vi "Insert Error.Record.vi"(8 "error in (no error)":errorcluster, 11 "Error":T1) -> (0 "error out":errorcluster)   [LabVIEW 2017, in "SQLite.lvclass"]
doc: "更新Limitation表格里面的Min和Max，根据输入的不同而更新不同的内容。\nValue 的输入必须最少包含Min和Max的值。\n\n2015-11-03 10:20:20\n蒋松\njiangsong@outlook.com"
uses:
  SQLite.lvclass
  Error Details.ctl
  SQLiteFileName.ctl
  TabelFullName.ctl
  <vilib>/Utility/error.llb/Trim Whitespace.vi
  <userlib>/sushu/sushu.lvlib
  <userlib>/LabSQL/LabSQL.lvlib
panel:
  in  "VI Ref":refnum<vi>
  in  "Alarm?":bool=TRUE
  in  "CMD":T2(ring)=enum."Read"
  out "array":string[](array[string])
  out "concatenated string":string
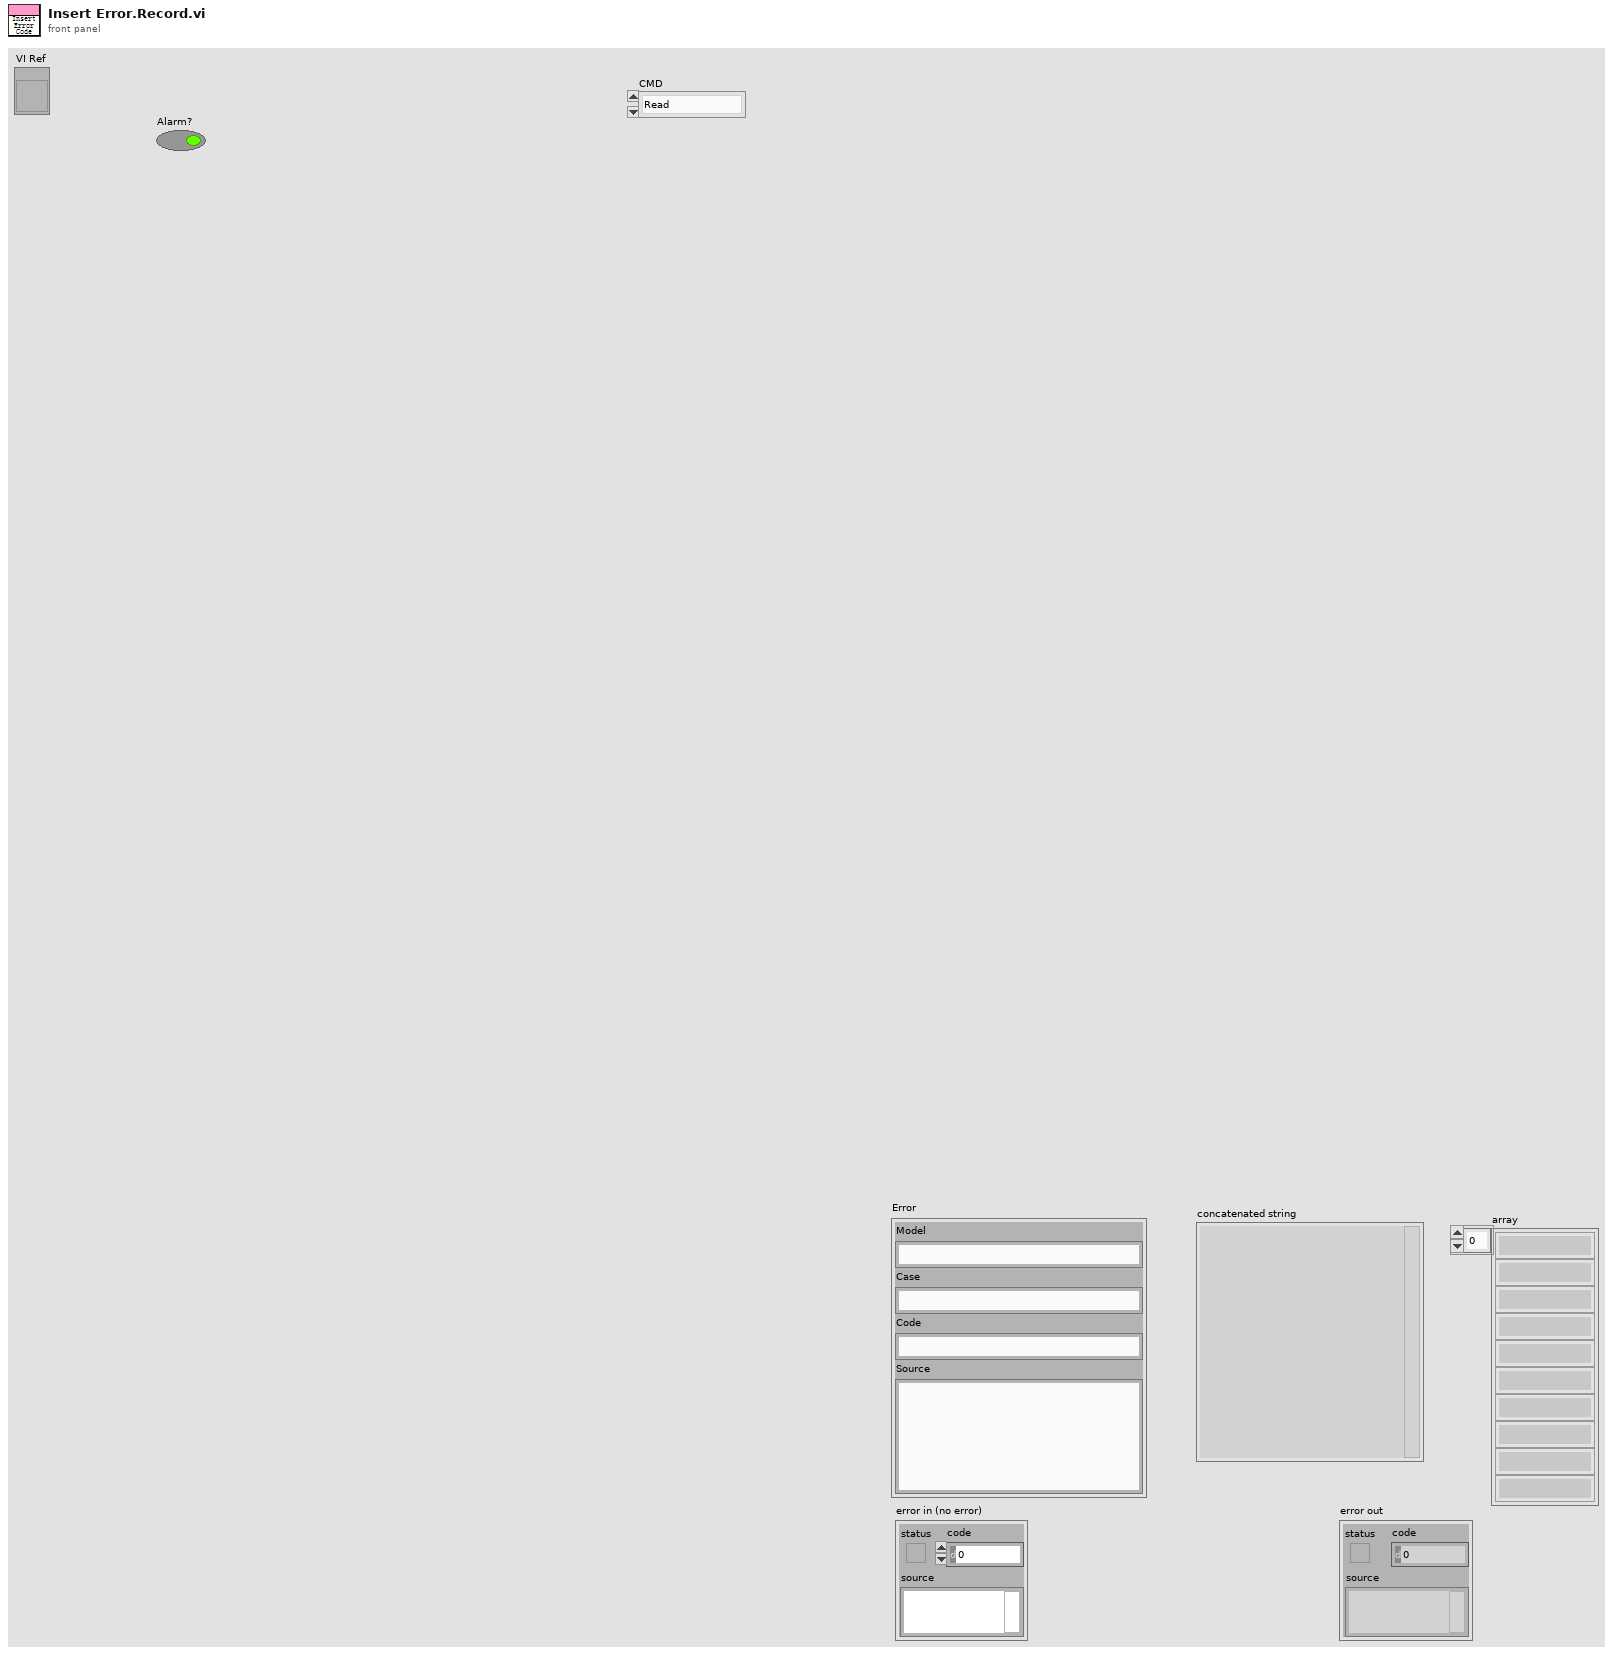
[diagram p1: front panel]
types:
  T1 = typedef "SQLite.lvclass/Error Details.ctl" = cluster{"Model":string, "Case":string, "Code":string, "Source":string}
  T2 = enum16{"Initialize", "Read", "Write", "UnInitialize"}
  T3 = typedef "SQLite.lvclass/TabelFullName.ctl" = string
  T4 = typedef "SQLite.lvclass/SQLiteFileName.ctl" = string
  T5 = cluster{"Current VI Reference":refnum<vi>, "Close Panel on Exit?":bool}
  T6 = cluster{"Core":cluster{"Current VI Reference":refnum<vi>, "Close Panel on Exit?":bool}, "VI Name":string}
  T7 = enum32{"invalid app kind", "Development System", "Run Time System", "Student Edition", "Embedded LabVIEW", "Evaluation", "Custom"}
  T8 = enum32{"Invalid", "Standard", "Closed", "Hidden", "Minimized", "Maximized"}
  T9 = enum16{"Other", "SQL2008", "SQLite", "Access", "MySQL"}
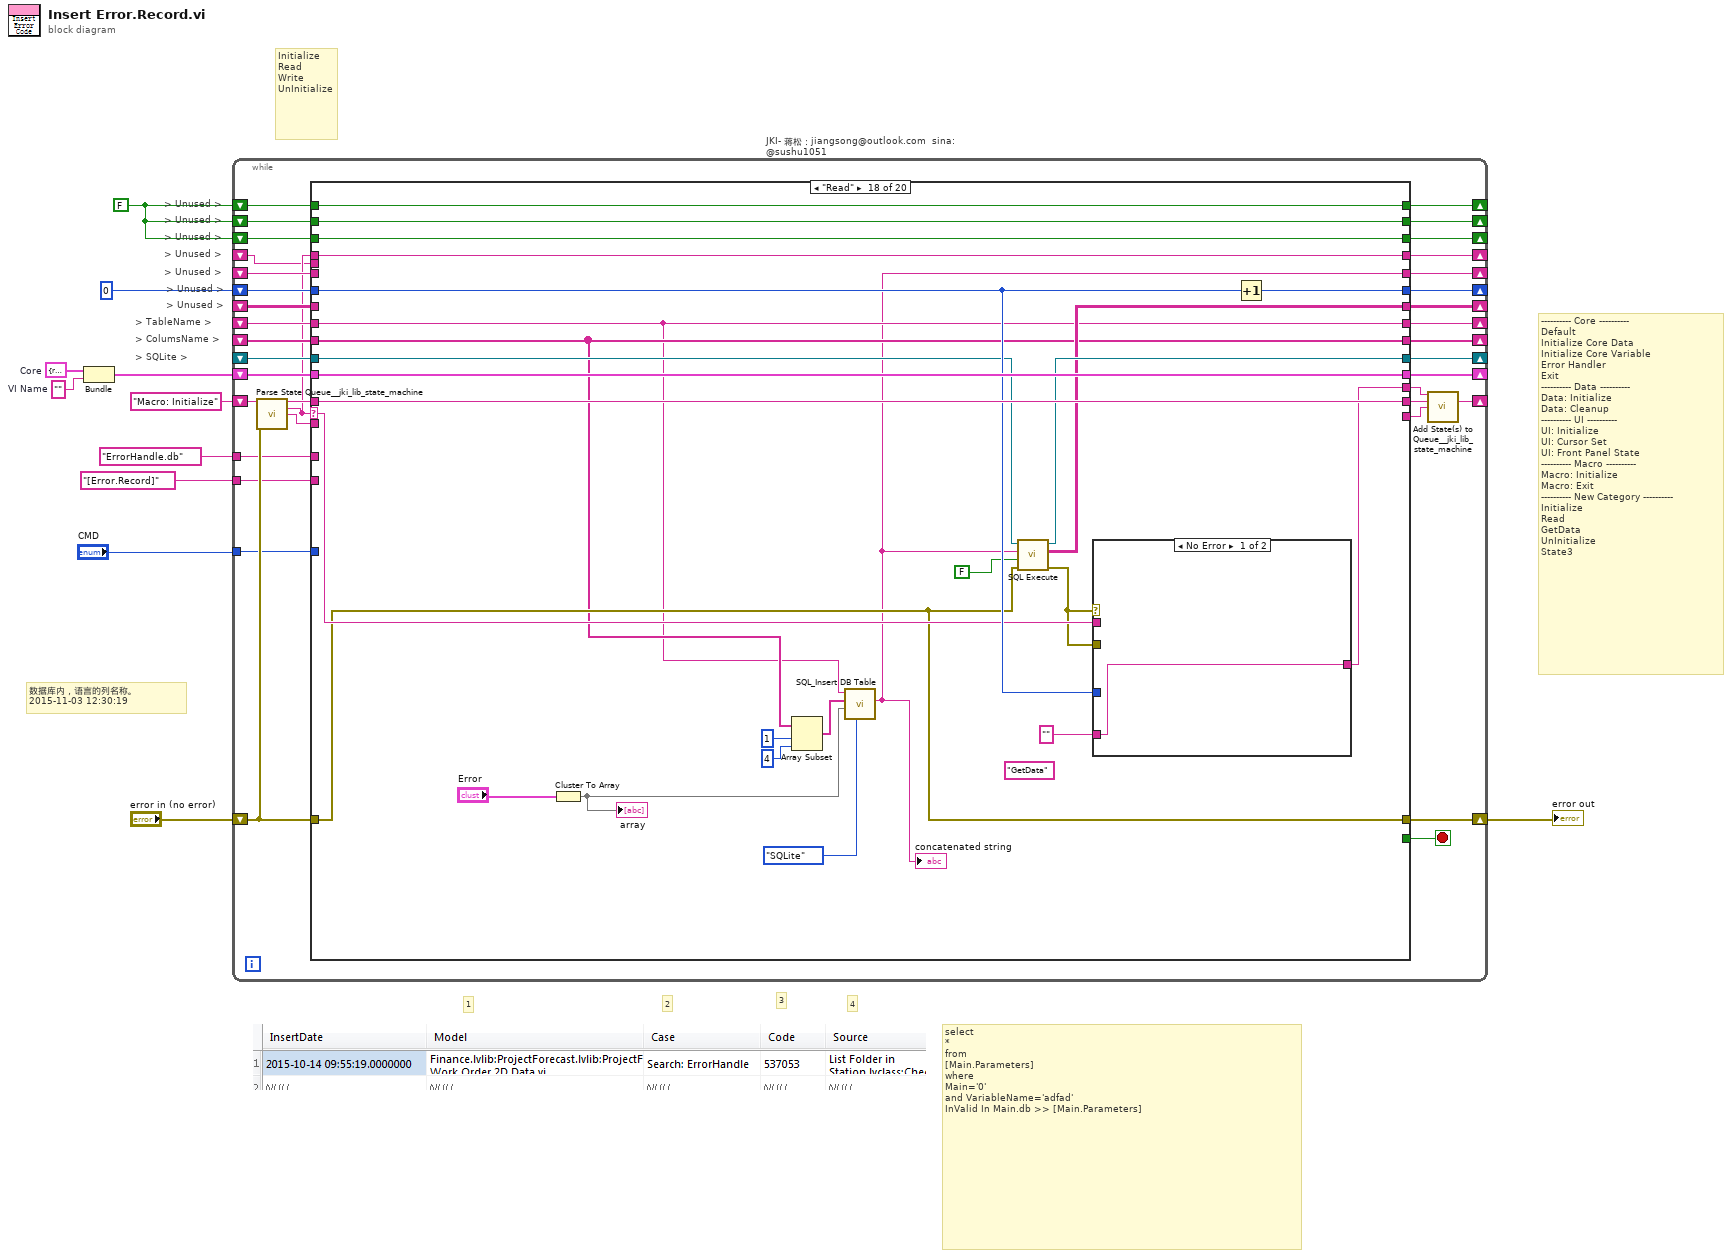
[diagram p0: block diagram]
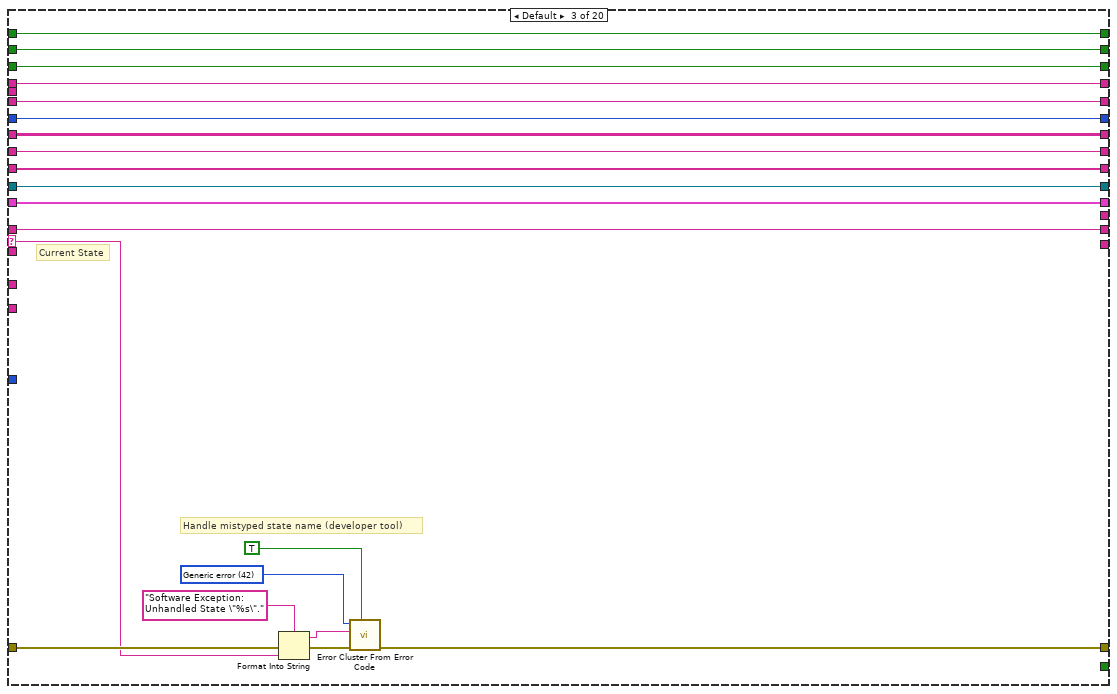
[diagram p4: hidden frame]
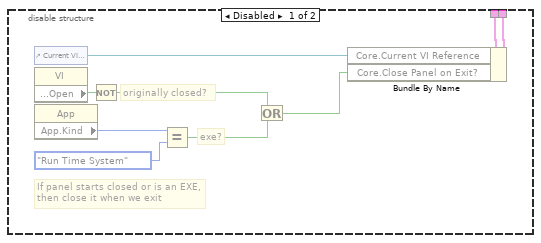
[diagram p6: hidden frame]
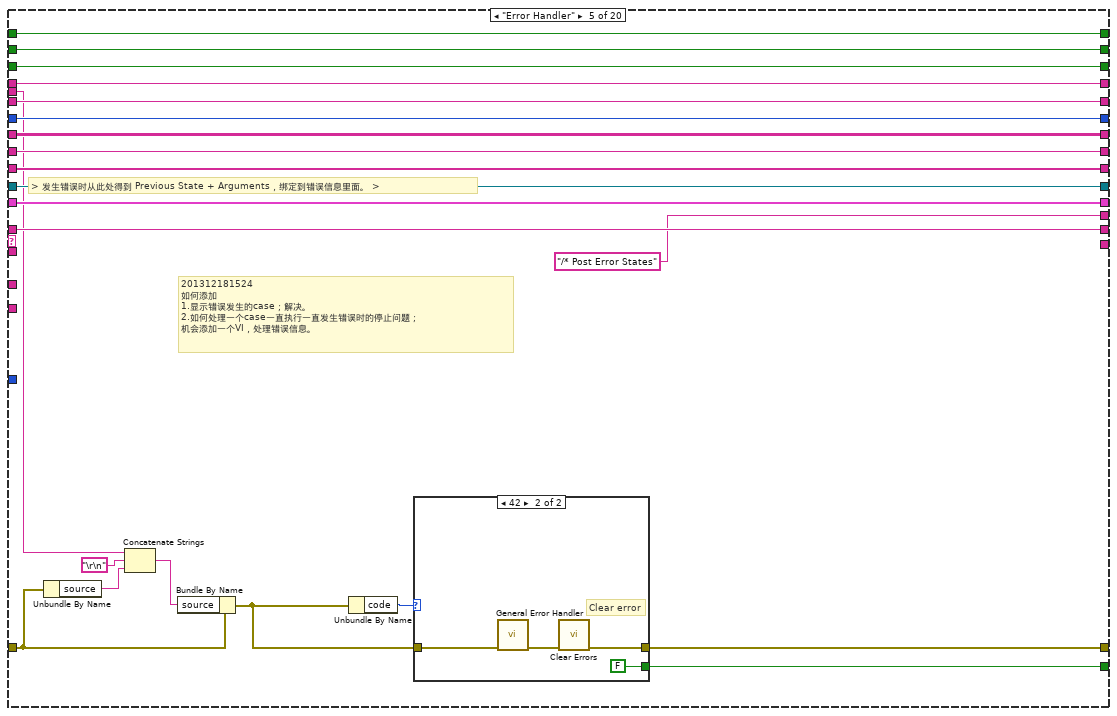
[diagram p7: hidden frame]
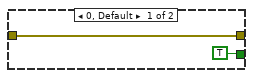
[diagram p8: hidden frame]
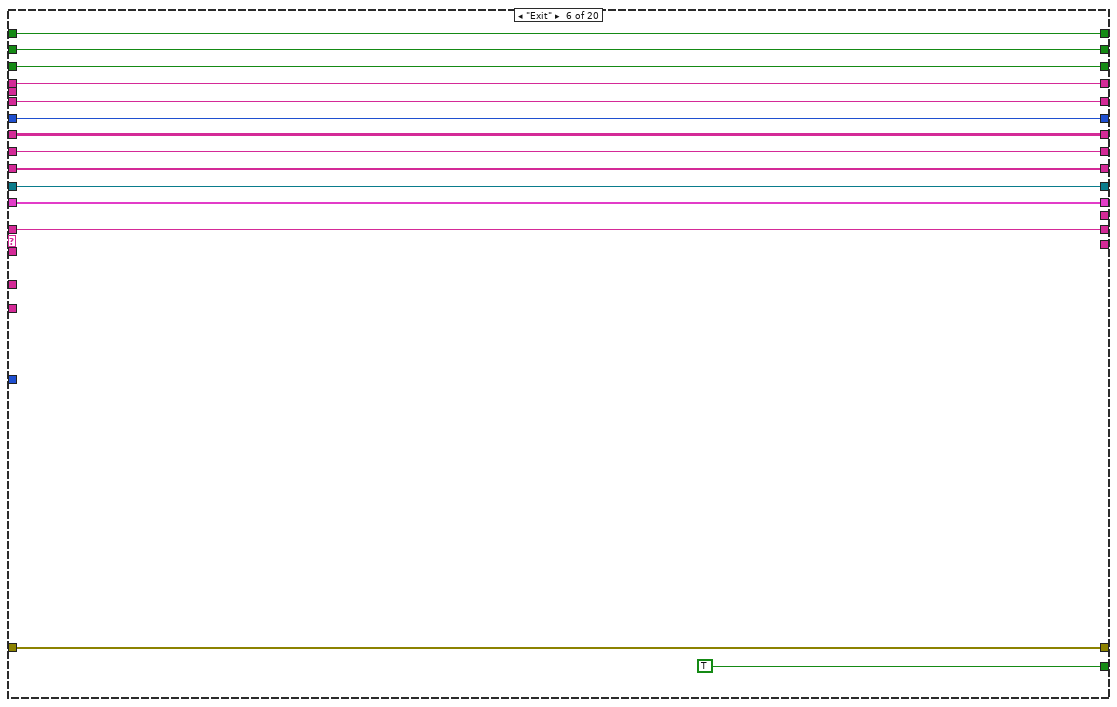
[diagram p9: hidden frame]
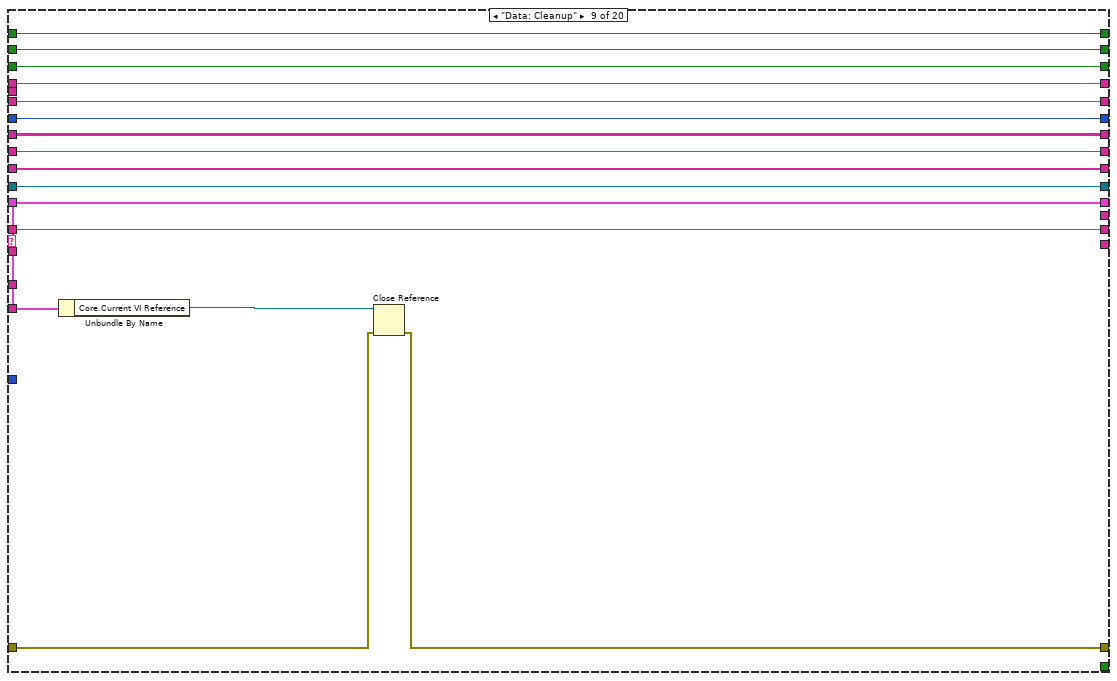
[diagram p12: hidden frame]
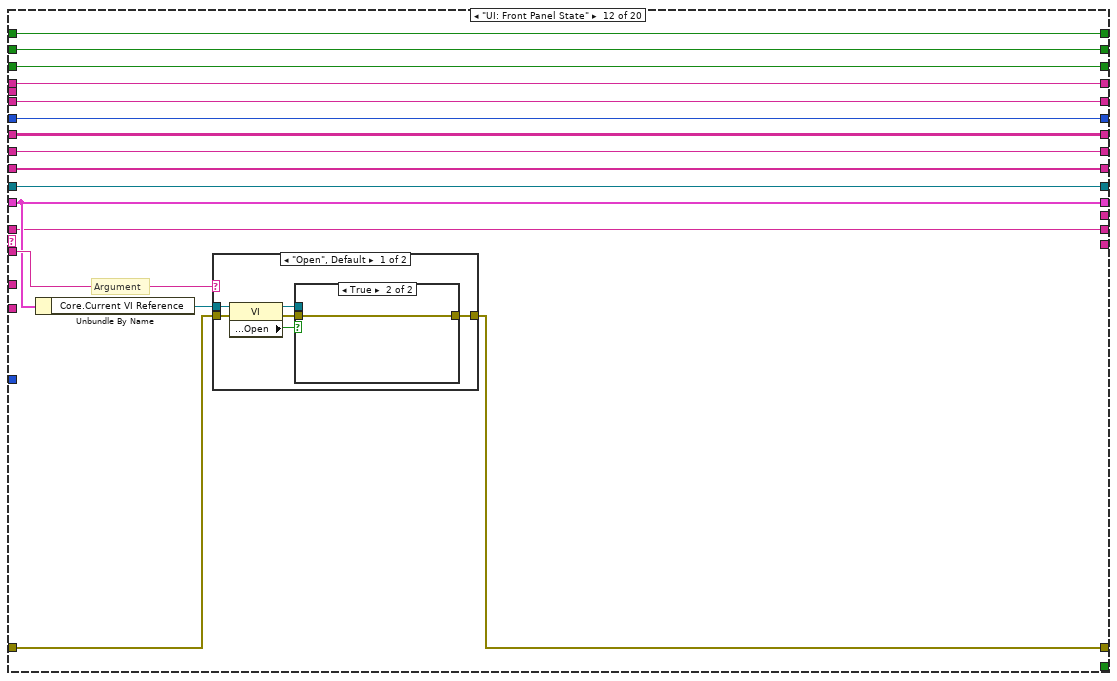
[diagram p15: hidden frame]
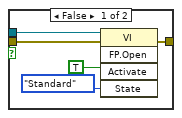
[diagram p16: hidden frame]
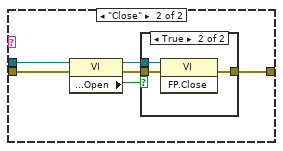
[diagram p17: hidden frame]
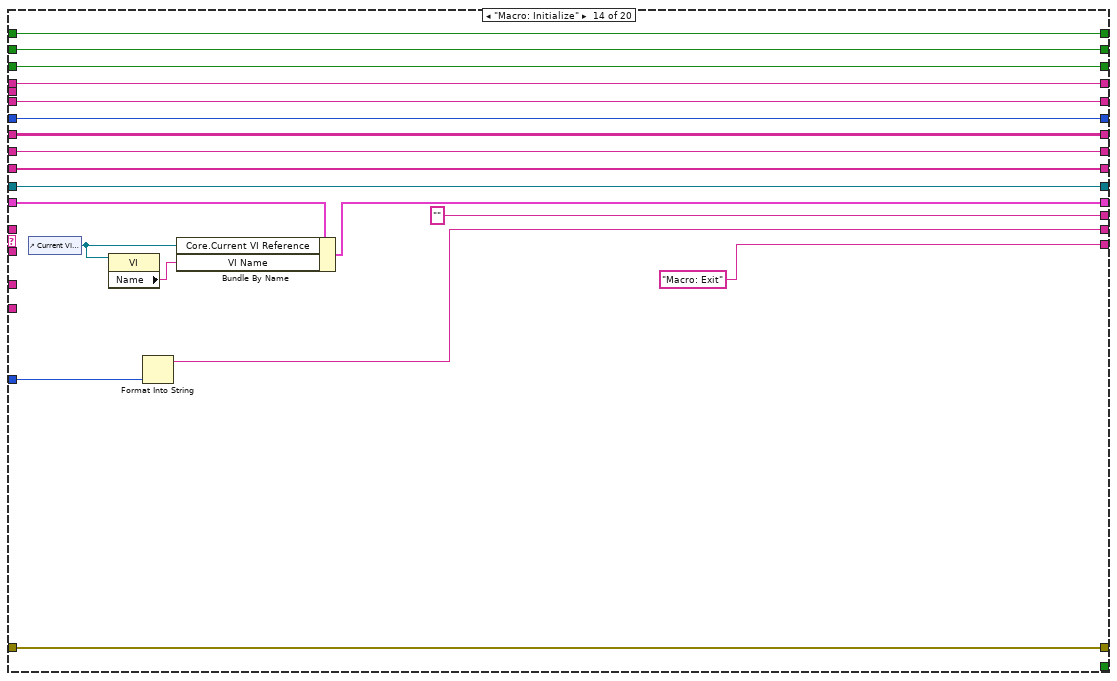
[diagram p20: hidden frame]
diagram:
  w11 = ""  # VI Name
  w10 = T5 {"Current VI Reference"=refnum, "Close Panel on Exit?"=FALSE}  # Core
  w5 = FALSE
  # "Initialize\nRead\nWrite\nUnInitialize"
  # "> Unused >"
  # "> Unused >"
  # "> Unused >"
  # "> Unused >"
  # "> Unused >"
  # "> Unused >"
  # "> SQLite >"
  # "> ColumsName >"
  # "> TableName >"
  # "> Unused >"
  # "---------- Core ----------\nDefault\nInitialize Core Data\nInitialize Core Variable\nError Handler\nExit\n---------- Data ----------\nData: Initialize\nData: Cleanup\n---------- UI ----------\nUI: Initialize\nUI: Cursor Set\nUI: Front Panel State\n---------- Macro ----------\nMacro: Initialize\nMacro: Exit\n---------- New Category ----------\nInitialize\nRead\nGetData\nUnInitialize\nState3"
  # "数据库内，语言的列名称。\n2015-11-03 12:30:19"
  # "4"
  # "3"
  # "2"
  # "1"
  # "select\n*\nfrom\n[Main.Parameters]\nwhere\nMain='0'\nand VariableName='adfad'\nInValid In Main.db >> [Main.Parameters]"
  n1 = Bundle("Core"=w10, "VI Name"=w11) -> (w9:T6)  [unwired: 1 in]
  n2 = while "JKI- 蒋松：jiangsong@outlook.com  sina: @sushu1051" {
    shift-right: [w45] -> w1
    shift-left: "error in (no error)" -> [w43]
    shift-right: [w32] -> _
    shift-left: "Macro: Initialize" -> [w33]
    shift-right: [w39] -> _
    shift-left: _ -> [w41]
    shift-right: [w40] -> _
    shift-left: _ -> [w42]
    shift-right: [w34] -> _
    shift-left: w9 -> [w37]
    shift-right: [w35] -> _
    shift-left: _ -> [w28]
    shift-right: [w36] -> _
    shift-left: _ -> [w38]
    shift-right: [w27] -> _
    shift-left: 0 -> [w26]
    shift-right: [w20] -> _
    shift-left: w5 -> [w18]
    shift-right: [w19] -> _
    shift-left: w5 -> [w17]
    shift-right: [w22] -> _
    shift-left: _ -> [w23]
    shift-right: [w21] -> _
    shift-left: _ -> [w12]
    shift-right: [w24] -> _
    shift-left: w5 -> [w25]
    tunnel: "CMD" -> [w16]
    tunnel: T4 "ErrorHandle.db" ("SQLiteFileName") -> [w15]
    tunnel: T3 "[Error.Record]" ("TabelFullName") -> [w14]
    stop <- w44 stop-if-true
    n3 = call <vilib>:"Parse State Queue__jki_lib_state_machine.vi"("State Queue"=w33, "Error In (no error)"=w43) -> ("Remaining States"=w47:string, "Current State"=w13:string, "Arguments"=w46:string)  [unwired: 10 in, 1 out]
    n4 = case shown="\"Read\"" w13 {
      selector: w13 -> [_ _ w81 _ _ _ _ _ _ _ _ _ _ _ _ _ _ w363 _ _]
      tunnel: w47 -> [w60 w67 w80 w100 w131 w152 w166 w180 w192 w207 w220 w233 w271 _ w304 w321 w347 w373 w403 w436]
      tunnel: w46 -> [_ _ _ _ _ _ _ _ _ _ _ w236 _ _ _ _ _ _ _ _]
      tunnel: [w59 w73 w82 w104 w125 w154 w168 w182 w194 w209 w222 w237 w273 w293 w311 w324 w328 w359 w388 w422] -> w45
      tunnel: w43 -> [w59 w73 w83 w104 w135 w154 w168 w182 w195 w209 w222 w238 w273 w293 w311 w324 w328 w359 w389 w423]
      tunnel: [w60 w67 w80 w100 w131 w152 w166 w180 w192 w207 w220 w233 w271 w279 w304 w321 w347 w373 w403 w436] -> w31
      tunnel: [_ _ _ _ w124 TRUE _ _ _ _ _ _ _ _ _ _ _ _ _ _] -> w44
      tunnel: w42 -> [w58 w72 w93 w107 w139 w159 w172 w185 w200 w213 w226 w242 w277 w296 w314 w327 w346 _ w390 w435]
      tunnel: w41 -> [w57 w71 w92 w106 w138 w158 w171 w184 w199 w212 w225 w241 w276 w295 w313 w326 _ w353 w402 w434]
      tunnel: [w58 w72 w93 w107 w139 w159 w172 w185 w200 w213 w226 w242 w277 w296 w314 w327 w346 w360 w390 w435] -> w40
      tunnel: [w57 w71 w92 w106 w138 w158 w171 w184 w199 w212 w225 w241 w276 w295 w313 w326 w329 w353 w402 w434] -> w39
      tunnel: w38 -> [w56 w70 w91 w105 w137 w157 w170 w183 w198 w211 w224 w240 w275 w294 w312 w325 _ w354 w401 w433]
      tunnel: w28 -> [w54 w68 w90 w101 w129 w153 w167 w181 w193 w208 w221 w234 w272 w292 w305 w322 _ w362 w400 w425]
      tunnel: w37 -> [w55 w69 w89 w103 w136 w156 w169 w173 w196 w210 w223 w235 w274 w281 w306 w323 w345 w372 w399 w432]
      tunnel: [w56 w70 w91 w105 w137 w157 w170 w183 w198 w211 w224 w240 w275 w294 w312 w325 w331 w354 w401 w433] -> w36
      tunnel: [w54 w68 w90 w101 w129 w153 w167 w181 w193 w208 w221 w234 w272 w292 w305 w322 w333 w361 w400 w424] -> w35
      tunnel: [w55 w69 w89 w102 w136 w156 w169 w173 w196 w210 w223 w235 w274 w280 w306 w323 w345 w372 w399 w432] -> w34
      tunnel: [_ _ _ _ "/* Post Error States" _ _ _ _ _ _ _ _ "" w303 _ _ w365 _ _] -> w30
      tunnel: [_ _ _ _ _ _ _ _ _ _ _ _ _ "Macro: Exit" _ _ _ _ _ _] -> w29
      tunnel: w26 -> [w53 w66 w79 w99 w128 w151 w165 w179 w191 w206 w219 w232 w270 w291 w302 w320 w344 w366 w398 w431]
      tunnel: [w53 w66 w79 w99 w128 w151 w165 w179 w191 w206 w219 w232 w270 w291 w302 w320 w344 w367 w398 w431] -> w27
      tunnel: w17 -> [w51 w64 w77 w97 w122 w149 w163 w177 w189 w204 w217 w230 w268 w287 w300 w318 w339 w370 w397 w430]
      tunnel: w18 -> [w50 w63 w76 w96 w121 w148 w162 w176 w188 w203 w216 w229 w267 w286 w299 w317 w340 w369 w396 w429]
      tunnel: [w51 w64 w77 w97 w122 w149 w163 w177 w189 w204 w217 w230 w268 w287 w300 w318 w339 w370 w397 w430] -> w19
      tunnel: [w50 w63 w76 w96 w121 w148 w162 w176 w188 w203 w216 w229 w267 w286 w299 w317 w340 w369 w396 w429] -> w20
      tunnel: w13 -> [w49 w62 w75 w95 w120 w147 w161 w175 w187 w202 w215 w228 w266 w285 w298 w316 w341 w368 w395 w428]
      tunnel: w23 -> [w48 w61 w74 w94 w119 w146 w160 w174 w186 w201 w214 w227 w265 w284 w297 w315 w342 _ w385 w427]
      tunnel: [w49 w62 w75 w95 w120 w147 w161 w175 w187 w202 w215 w228 w266 w285 w298 w316 w341 w368 w395 w428] -> w21
      tunnel: [w48 w61 w74 w94 w119 w146 w160 w174 w186 w201 w214 w227 w265 w284 w297 w315 w342 w351 w385 w427] -> w22
      tunnel: w25 -> [w52 w65 w78 w98 w123 w150 w164 w178 w190 w205 w218 w231 w269 w288 w301 w319 w343 w371 w394 w426]
      tunnel: [w52 w65 w78 w98 w123 w150 w164 w178 w190 w205 w218 w231 w269 w288 w301 w319 w343 w371 w394 w426] -> w24
      tunnel: w16 -> [_ _ _ _ _ _ _ _ _ _ _ _ _ w278 _ _ _ _ _ _]
      tunnel: w15 -> [_ _ _ _ _ _ _ _ _ _ _ _ _ _ _ _ w332 _ w387 _]
      tunnel: w14 -> [_ _ _ _ _ _ _ _ _ _ _ _ _ _ _ _ w330 _ w386 _]
      tunnel: w12 -> [_ _ _ _ w118 _ _ _ _ _ _ _ _ _ _ _ _ _ _ _]
      frame "Idle" {
      }
      frame "---------- Core ----------" {
      }
      frame Default {
        w85 = 42 items=["No error", "Argument error", "Memory is full", "Out of zone", "End of file", "File already open", "Generic file I/O error", "File not found", "File permission error", "Disk is full", "Duplicate path", "Too many files open", "System feature not enabled", "Resource file not found", "Cannot add resource", "Resource not found", "Image not found", "Image memory error", "Pen does not exist", "Config type invalid", "Config token not found", "Config parse error", "Config memory error", "Bad external code format", "Bad external code offset", "External code not present", "Null window", "Destroy window error", "Null menu", "Print aborted", "Bad print record", "Print driver error", "Windows error during printing", "Memory error during printing", "Print dialog error", "Generic print error", "Invalid device refnum", "Device not found", "Device parameter error", "Device unit error", "Cannot open device", "Device call aborted", "Generic error", "Cancelled by user", "Object ID too low", "Object ID too high", "Object not in heap", "Unknown heap", "Unknown object (invalid DefProc)", "Unknown object (DefProc not in table)", "Message out of range", "Invalid (null) method", "Unknown message", "Manager call not supported", "Bad address", "Network operation in progress", "Network operation timed out", "Connection is busy", "Network attribute not supported", "Network error", "Address in use", "System out of memory", "Connection aborted", "Connection refused", "Not connected", "Already connected", "Connection closed", "Initialization error (interapplication manager)", "Bad occurrence", "Wait on unbound occurrence handler", "Occurrence queue overflow", "Datalog type conflict", "Unused", "Unrecognized type (interapplication manager)", "Memory corrupt", "Failed to make temporary DLL", "Old CIN version", "Drag socket not found", "Failed to load drop-object", "Failed to register OLE object", "Failed to release OLE object", "Format specifier type mismatch", "Unknown format specifier", "Too few format specifiers", "Too many format specifiers", "Scan failed", "Newer CIN version", "Error converting to variant", "Runtime menu error", "Password tampered", "Variant attribute not found", "Incompatible variant data type", "Event data is not available", "Event Store is not present", "Occurrence is not found", "Event Queue is not created", "Event info is not available", "Refnum passed is NULL", "Error retrieving Class GUID", "Error retrieving CoClass GUID", "Error retrieving TypeLib GUID.", "Bad built application magic bytes.", "Specific driver is different from the specific driver associated with the Logical Name.", "There is no session opened to the class driver.", "Max Error", "MAX - Error with config objects", "MAX - Error loading configuration", "MAX - Group not supported"]
        # "Current State"
        # "Handle mistyped state name (developer tool)"
        n5 = Format Into String(format string="Software Exception: Unhandled State \"%s\"." ("message"), error in=w83, w81) -> (resulting string=w86:string, error out=w87:errorcluster)  [unwired: 1 in]
        n6 = call <vilib>:"Error Cluster From Error Code.vi"("show call chain? (False)"=TRUE, "error in (no error)"=w87, "error message (\"\")"=w86, "error code (0)"=w85) -> ("error out"=w82:errorcluster)  [unwired: 5 in]
      }
      frame "Initialize Core Data" {
        n7 = disable-structure shown="Enabled" {
          disable-tunnel: w103 -> [w109 w117]
          disable-tunnel: [w108 w117] -> w102
          frame Disabled {
            # "originally closed?"
            # "exe?"
            # "If panel starts closed or is an EXE, then close it when we exit"
            n8 = control-ref of="Current VI Reference"() -> (w116:refnum<vi>)
            n9 = property class="VI"() -> ("Front Panel.Open"=w110:bool)  [unwired: 2 in, 2 out]
            n10 = property class="App"() -> ("App.Kind"=w111:T7)  [unwired: 2 in, 2 out]
            n11 = Not(x=w110) -> (.not. x?=w113:bool)
            n12 = Equal?(x=w111, y=T7."Run Time System" ("Application:Kind")) -> (x = y?=w114:bool)
            n13 = Or(x=w113, y=w114) -> (x .or. y?=w115:bool)
            n14 = Bundle By Name(cluster=w109, "Core.Current VI Reference"=w116, "Core.Close Panel on Exit?"=w115) -> (w108:T6)
          }
          frame Enabled {
          }
        }
      }
      frame "Error Handler" {
        # "> 发生错误时从此处得到 Previous State + Arguments，绑定到错误信息里面。 >"
        # "201312181524\n如何添加\n1.显示错误发生的case；解决。\n2.如何处理一个case一直执行一直发生错误时的停止问题；\n机会添加一个VI，处理错误信息。"
        # "Clear error"
        n15 = Unbundle By Name(w135) -> ("source"=w133:string)
        n16 = Concatenate Strings(w118, "\r\n", w133) -> (w132:string)
        n17 = Bundle By Name(cluster=w135, "source"=w132) -> (w126:errorcluster)
        n18 = Unbundle By Name(w126) -> ("code"=w127:i32)
        n19 = case shown="42" w127 {
          tunnel: [TRUE FALSE] -> w124
          tunnel: w126 -> [w141 w144]
          tunnel: [w141 w142] -> w125
          frame 0, Default {
          }
          frame 42 {
            n20 = call <vilib>:"General Error Handler.vi"("error in (no error)"=w144) -> ("error out"=w143:errorcluster)  [unwired: 10 in, 4 out]
            n21 = call <vilib>:"Clear Errors.vi"("error in (no error)"=w143) -> ("error out"=w142:errorcluster)  [unwired: 5 in, 1 out]
          }
        }
      }
      frame "Exit" {
      }
      frame "---------- Data ----------" {
      }
      frame "Data: Initialize" {
      }
      frame "Data: Cleanup" {
        n22 = Unbundle By Name(w196) -> ("Core.Current VI Reference"=w197:refnum<vi>)
        n23 = Close Reference(reference=w197, error in (no error)=w195) -> (error out=w194:errorcluster)
      }
      frame "---------- UI ----------" {
      }
      frame "UI: Initialize" {
      }
      frame "UI: Front Panel State" {
        # "Argument"
        n24 = Unbundle By Name(w235) -> ("Core.Current VI Reference"=w239:refnum<vi>)
        n25 = case shown="\"Open\", Default" w236 {
          tunnel: w238 -> [w246 w259]
          tunnel: [w248 w260] -> w237
          tunnel: w239 -> [w247 w257]
          frame "Open", Default {
            n26 = property class="VI"(reference=w247, error in=w246) -> (reference out=w244:refnum<vi>, error out=w245:errorcluster, "Front Panel.Open"=w243:bool)
            n27 = case shown="True" w243 {
              tunnel: [w251 w254] -> w248
              tunnel: w245 -> [w250 w254]
              tunnel: w244 -> [w249 _]
              frame False {
                n28 = invoke class="VI" method="FP.Open"(reference=w249, error in=w250, "Activate"=TRUE, "State"=T8."Standard") -> (error out=w251:errorcluster)  [unwired: 1 in, 4 out]
              }
              frame True {
              }
            }
          }
          frame "Close" {
            n29 = property class="VI"(reference=w257, error in=w259) -> (reference out=w256:refnum<vi>, error out=w258:errorcluster, "Front Panel.Open"=w255:bool)
            n30 = case shown="True" w255 {
              tunnel: [w261 w264] -> w260
              tunnel: w258 -> [w261 w263]
              tunnel: w256 -> [_ w262]
              frame False {
              }
              frame True {
                n31 = invoke class="VI" method="FP.Close"(reference=w262, error in=w263) -> (error out=w264:errorcluster)  [unwired: 1 in, 2 out]
              }
            }
          }
        }
      }
      frame "---------- Macro ----------" {
      }
      frame "Macro: Initialize" {
        n32 = control-ref of="Current VI Reference"() -> (w282:refnum<vi>)
        n33 = property class="VI"(reference=w282) -> ("Name"=w283:string)  [unwired: 1 in, 2 out]
        n34 = Format Into String(w278) -> (resulting string=w279:string)  [unwired: 3 in, 1 out]
        n35 = Bundle By Name(cluster=w281, "Core.Current VI Reference"=w282, "VI Name"=w283) -> (w280:T6)
      }
      frame "Macro: Exit" {
        n36 = Unbundle By Name(w306) -> ("Core.Close Panel on Exit?"=w307:bool)
        n37 = Select(t="UI: Front Panel State >> Close", s=w307, f="") -> ()  [unwired: 1 out]
        n38 = call <vilib>:"Add State(s) to Queue__jki_lib_state_machine.vi"("State(s) at Back (\"\")"="Data: Cleanup\nExit") -> ("States Out"=w303:string)  [unwired: 14 in]
      }
      frame "---------- New Category ----------" {
      }
      frame "Initialize" {
        n39 = Concatenate Strings(w330) -> (w329:string)
        n40 = call "SQLite File Path.vi"("SQLiteFileName"=w332, "SQLite in"=refnum<class "SQLite.lvclass"> refnum ("SQLite.lvclass")) -> ("string"=w336:string, "SQLite out"=w338:refnum<class "SQLite.lvclass">)  [unwired: 7 in, 1 out]
        n41 = call-dynamic "Open Connection.vi"("ConnectionString"=w336, "HostDB in"=w338) -> ("error out"=w335:errorcluster, "HostDB out"=w334:refnum<class "SQLite.lvclass">)  [unwired: 8 in]
        n42 = call-dynamic "Get Table Columns Name.vi"("error in (no error)"=w335, "TableName"=w329, "HostDB in"=w334) -> ("ColunmsList"=w331:string[], "HostDB out"=w333:refnum<class "SQLite.lvclass">)  [unwired: 4 in, 3 out]
      }
      frame "Read" {
        (unwired) "GetData" ("f")
        n43 = Cluster To Array(cluster="Error") -> (array=w352:string[])
        "array" <- w352
        n44 = Array Subset(array=w354, index=1, length=4) -> (w356:string[])
        n45 = call <userlib>:"SQL_Insert DB Table.vi"("DB Type"=T9."SQLite", "ColumnsValue"=w352, "ColumnsName"=w356, "Table Name"=w353) -> ("Insert DB String"=w351:string)  [unwired: 7 in]
        "concatenated string" <- w351
        n46 = call-dynamic "SQL Execute.vi"("error in (no error)"=w359, "Return Data (T)"=FALSE, "Command Text"=w351, "HostDB in"=w362) -> ("error out"=w358:errorcluster, "Table Control"=w360:string[][], "HostDB out"=w361:refnum<class "SQLite.lvclass">)  [unwired: 3 in, 2 out]
        n47 = case shown="No Error" w358 {
          tunnel: w358 -> [_ w384]
          tunnel: w366 -> [_ w383]
          tunnel: [w374 w380] -> w365
          tunnel: "" ("f") -> [w374 w379]
          tunnel: w363 -> [_ w376]
          frame No Error {
          }
          frame Error {
            n48 = Unbundle By Name(w384) -> ("status"=w375:bool)
            n49 = Equal To 0?(x=w383) -> (x = 0?=w382:bool)
            n50 = And(x=w375, y=w382) -> (x .and. y?=w381:bool)
            n51 = call <vilib>:"Add State(s) to Queue__jki_lib_state_machine.vi"("State(s) in Front (\"\")"="Initialize" ("Remaining States"), "State(s) in (\"\")"=w376) -> ("States Out"=w377:string)  [unwired: 13 in]
            n52 = Select(t=w377, s=w381, f=w379) -> (s? t:f=w380:string)
          }
        }
        n53 = Increment(x=w366) -> (x+1=w367:i32)
      }
      frame "GetData" {
        n54 = Empty Array?(array=w390) -> (empty?=w392:bool)
        n55 = And(x=w392, y="Alarm?") -> (x .and. y?=w393:bool)
        n56 = case shown="False" w393 {
          tunnel: [w407 w420] -> w388
          tunnel: w389 -> [w407 w421]
          tunnel: w385 -> [_ w417]
          tunnel: w387 -> [_ w419]
          tunnel: w386 -> [_ w418]
          tunnel: w390 -> [w404 _]
          frame False {
            w405 = 0 ("index (row)")
            # "DBL 和 字符串 都输出，需要那个用那个。\n2015-11-03 10:44:12\n蒋松"
            n57 = Index Array(array=w404, index (row)=w405, index (col)=w405) -> ()  [unwired: 1 out]
            n58 = Index Array(array=w404, index (col)=0 ("disabled index (col)")) -> ()  [unwired: 1 in, 1 out]
          }
          frame True {
            n59 = Concatenate Strings(w419) -> (w416:string)
            n60 = Concatenate Strings(w418) -> (w415:string)
            n61 = call <vilib>:"Build State String with Arguments__JKI_lib_State_Machine.vi"("Arguments (\"\")"=w415, "State"=w416) -> ("State with Arguments"=w413:string)  [unwired: 4 in]
            n62 = Concatenate Strings(w417, "InValid In " ("Message"), w413) -> (w412:string)
            n63 = call <userlib>:"Errors Handle Dialoge.vi"("VI Ref"="VI Ref", "Cancel Text"="Ignore", "OK Text"="OK", "error in (no error)"=w421, "Title Text"="Select VariableName!", "Message"=w412) -> ("error out"=w420:errorcluster)  [unwired: 4 in, 1 out]
          }
        }
      }
      frame "UnInitialize" {
        n64 = call-dynamic "Close Connection.vi"("error in (no error)"=w423, "HostDB in"=w425) -> ("error out"=w422:errorcluster, "HostDB out"=w424:refnum<class "SQLite.lvclass">)  [unwired: 8 in]
      }
    }
    n65 = call <vilib>:"Add State(s) to Queue__jki_lib_state_machine.vi"("State(s) in Front (\"\")"=w30, "State(s) in (\"\")"=w31, "State(s) at Back (\"\")"=w29) -> ("States Out"=w32:string)  [unwired: 12 in]
  }
  "error out" <- w1
